vi "Matrix_IsEqual.vi"(9 "Tolerance":dbl=1e-06, 10 "other":T1, 11 "input matrix":T1) -> (3 "Equal":bool)   [LabVIEW 2019, in "Trajectory_Library.lvlib"]
doc: "Checks if another {@link Matrix} is equal to \"this\" within a specified tolerance.\n \nThis will check if each element is in tolerance of the corresponding element from the other Matrix.\n \n \nInputs:\n - input matrix -- The input matrix\n - other -- The matrix to check against this one.\n - tolerance -- The tolerance to check equality with. (Default is 1E-6)\n\nOutputs:\n - equal -- true if this matrix is equal to the one supplied."
uses:
  Trajectory_Library.lvlib
  <vilib>/Analysis/Matrix/Datatypes/RealMatrix.ctl
  <vilib>/Analysis/Matrix/NI_Matrix.lvlib
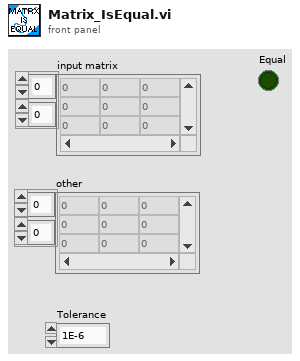
[diagram p1: front panel]
types:
  T1 = typedef "NI_Matrix.lvlib/RealMatrix.ctl" = dbl[][]
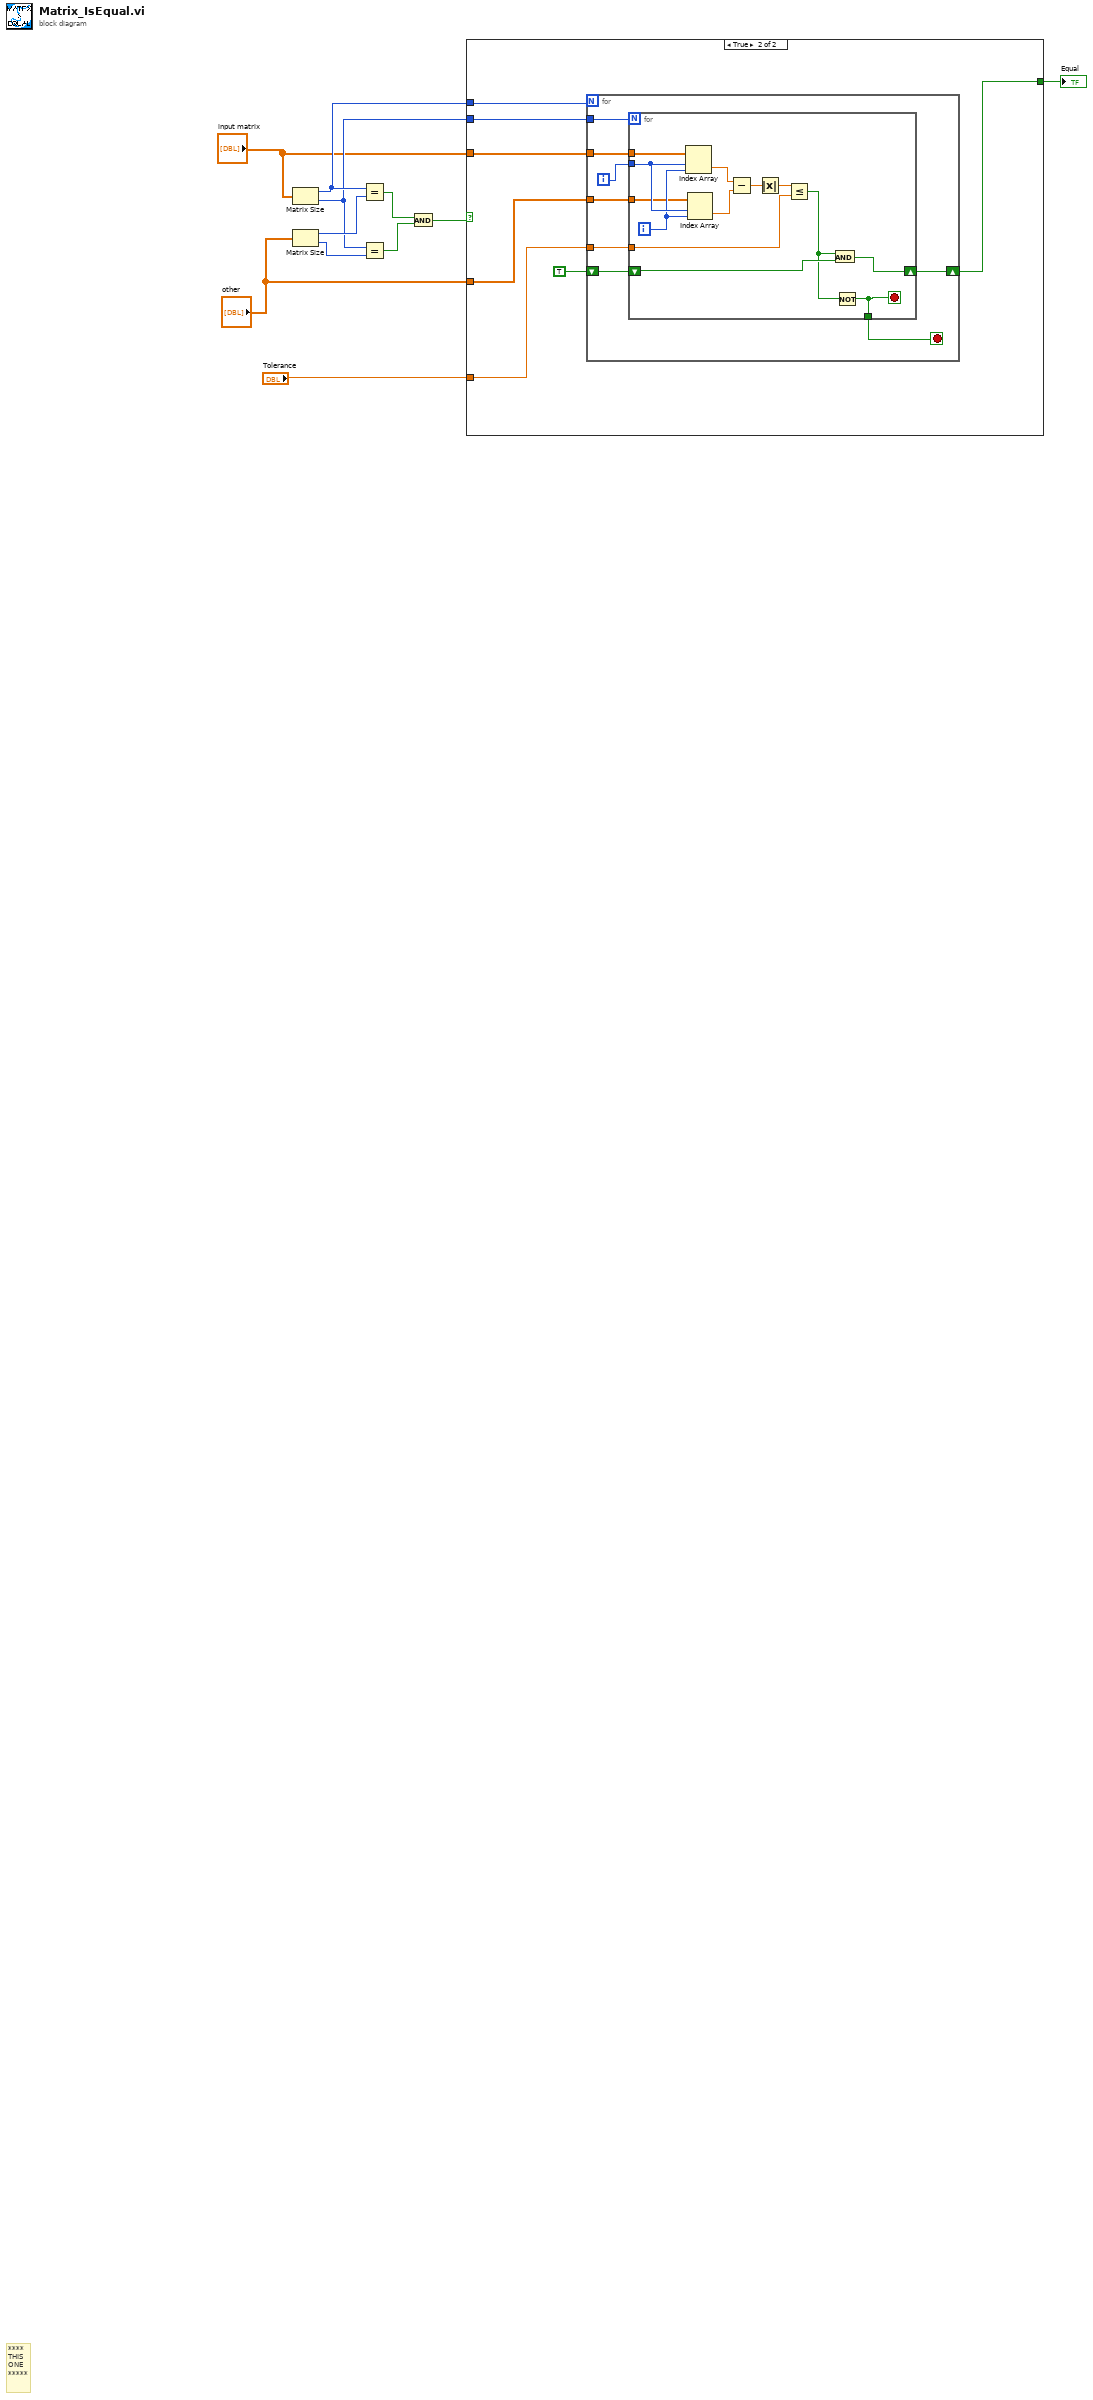
[diagram p0: block diagram]
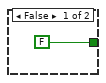
[diagram p2: hidden frame]
diagram:
  # "****\nTHIS\nONE\n*****"
  n1 = Matrix Size(0:"input matrix") -> (1:w5:i32, 2:w4:i32)
  n2 = Matrix Size(0:"other") -> (1:w11:i32, 2:w10:i32)
  n3 = Equal?(x=w5, y=w11) -> (x = y?=w9:bool)
  n4 = Equal?(x=w4, y=w10) -> (x = y?=w8:bool)
  n5 = And(x=w9, y=w8) -> (x .and. y?=w7:bool)
  n6 = case shown="True" w7 {
    tunnel: [FALSE w13] -> w6
    tunnel: w5 -> [_ w19]
    tunnel: w4 -> [_ w18]
    tunnel: "input matrix" -> [_ w17]
    tunnel: "other" -> [_ w16]
    tunnel: "Tolerance" -> [_ w15]
    frame False {
    }
    frame True {
      n7 = for {
        N: w19 -> [_]
        tunnel: w18 -> [w27]
        tunnel: w17 -> [w25]
        tunnel: w16 -> [w24]
        tunnel: w15 -> [w23]
        shift-right: [w20] -> w13
        shift-left: TRUE -> [w22]
        i -> [w26]
        stop <- w21 stop-if-true
        n8 = for {
          N: w27 -> [_]
          tunnel: w26 -> [w40]
          tunnel: w25 -> [w38]
          tunnel: w24 -> [w37]
          tunnel: w23 -> [w32]
          shift-right: [w28] -> w20
          shift-left: w22 -> [w31]
          tunnel: [w29] -> w21
          i -> [w39]
          stop <- w29 stop-if-true
          n9 = Index Array(array=w38, index (row)=w40, index (col)=w39) -> (element=w35:dbl)
          n10 = Index Array(array=w37, index (row)=w40, index (col)=w39) -> (element=w36:dbl)
          n11 = Subtract(x=w35, y=w36) -> (x-y=w34:dbl)
          n12 = Absolute Value(x=w34) -> (abs(x)=w33:dbl)
          n13 = Less Or Equal?(x=w33, y=w32) -> (x <= y?=w30:bool)
          n14 = And(x=w30, y=w31) -> (x .and. y?=w28:bool)
          n15 = Not(x=w30) -> (.not. x?=w29:bool)
        }
      }
    }
  }
  "Equal" <- w6
